vi "F5xxx_set_waveform.vi"(8 "error in":errorcluster, 9 "waveform string":string, 10 "waveform":enum16{"SINE", "TRI", "SQUARE"}(ring), 11 "VISA in":refnum<visa-resource-name>) -> (0 "error out":errorcluster, 3 "VISA out":refnum<visa-resource-name>)   [LabVIEW 2013]
panel:
  out "resulting string":string
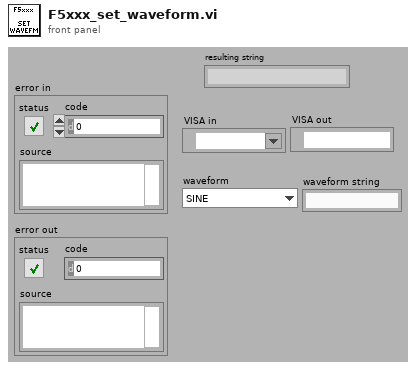
[diagram p1: front panel]
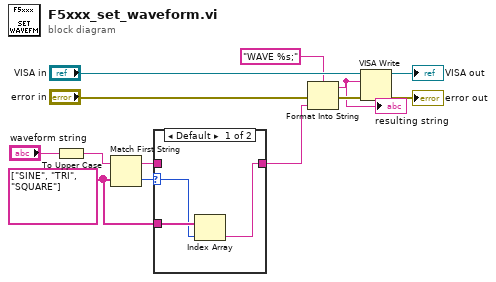
[diagram p0: block diagram]
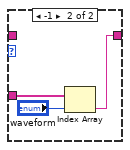
[diagram p2: hidden frame]
diagram:
  w6 = string[] ["SINE", "TRI", "SQUARE"] ("string array")
  n1 = To Upper Case(1:"waveform string") -> (0:w11:string)
  n2 = Match First String(2:w6, 3:w11) -> (0:w10:i32, 1:w9:string)
  n3 = case shown="Default" w10 {
    selector: w10 -> [w15 _]
    tunnel: w9 -> [_ _]
    tunnel: w6 -> [w16 w18]
    tunnel: [w14 w17] -> w2
    frame Default {
      n4 = Index Array(array=w16, index=w15) -> (element=w14:string)
    }
    frame -1 {
      n5 = Index Array(array=w18, index="waveform") -> (element=w17:string)
    }
  }
  n6 = Format Into String(format string="WAVE %s;", error in="error in", w2) -> (resulting string=w3:string, error out=w5:errorcluster)  [unwired: 1 in]
  "resulting string" <- w3
  n7 = VISA Write(VISA resource name="VISA in", write buffer=w3, error in (no error)=w5) -> (VISA resource name out=→"VISA out":refnum<visa-resource-name>, error out=→"error out":errorcluster)  [unwired: 1 out]
